vi "LuaVIEW Open.vi"(11 "error in (no error)":errorcluster) -> (6 "LuaVIEW reference":T1, 15 "error out":errorcluster)   [LabVIEW 2012]
doc: "Open a LuaVIEW state that can call public and export functions as well as the other types of LuaVIEW function. The resulting state (passed via the LuaVIEW reference) is ready for script compilation and subsequent execution. Once the LuaVIEW reference is no longer required, close it using \"LuaVIEW Close\" to free the associated resources.\n\nWhen the public function registry is not yet initialized and the \"auto-init registry\" global is set, the registry will be initialized first with all LuaVIEW function VIs in the built executable or, when running under development mode, with all LuaVIEW function VIs in the functions directory of the LuaVIEW toolkit.\n\nNote that the LuaVIEW reference returned by this VI is associated with a new and unique Lua state which entails an instance of the Lua virtual machine as well as the data space involved in compiling scripts and executing the resulting bytecode on that virtual machine instance. Scripts that run on different Lua states therefore have separate variable spaces."
uses:
  typedefs/t_LuaVIEW Reference.ctl
  typedefs/et_LuaVIEW CIN Actions.ctl
  typedefs/t_LuaVIEW CIN Spinlocked Actions.ctl
  glb_LuaVIEW Configuration Globals.vi
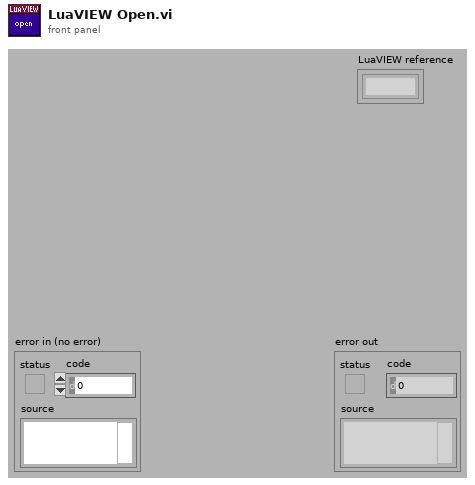
[diagram p1: front panel]
types:
  T1 = typedef "t_LuaVIEW Reference.ctl" = refnum<k1>
  T2 = typedef "et_LuaVIEW CIN Actions.ctl" = enum16{"checksynopsis", "_open", "_registerpublic", "_registerexport", "__never_an_error_result_ns", "luaversion", "cinversion", "_totals", "_taskcount", "pathological", "_unregnextpublic", "registryusecount", "__per_state_actions", "regsetprivate", "regsetindex", "regsetmodule", "_revokeexports", "_usepublic", "prepare", "compile", "execute", "call", "unregstaterefs", "_close", "pullboolean", "pullnumber", "pullI8", "pullU8", "pullI16", "pullU16", "pullI32", "pullU32", "pullobject", "pullrefnum", "pullstring", "pullflat", "pushflat", "pushobject", "getattribute", "setattribute", "stacktostring", "_startyieldtest", "_endyieldtest", "_pollprintbuffer", "__never_an_error_result_ps", "_pollexport", "setclone", "forcecleanup", "gettop", "clearstack", "insert", "pushboolean", "pushnumber", "pushrefnum", "pushstring", "pushnil", "pushvalue", "gettaskref", "settaskref"}
  T3 = typedef "t_LuaVIEW CIN Spinlocked Actions.ctl" = enum16{"totals", "taskcount", "open", "registerpublic", "registerexport", "revokeexports", "unregnextpublic", "usepublic", "pollexport", "close", "startyieldtest", "endyieldtest", "pollprintbuffer"}
  T4 = typedef "et_LuaVIEW CIN Results.ctl" = enum16{"OK", "error", "main", "call", "clonecall", "modulecall", "exportcall", "index", "yield"}
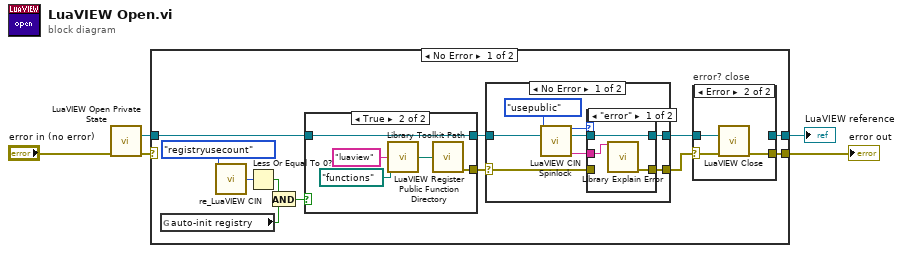
[diagram p0: block diagram]
diagram:
  n1 = call "LuaVIEW Open Private State.vi"("error in (no error)"="error in (no error)") -> ("LuaVIEW reference"=w1:T1, "error out"=w2:errorcluster)  [unwired: 13 in]
  n2 = case shown="No Error" w2 {
    selector: w2 -> [_ w45]
    tunnel: [w17 w44] -> w5
    tunnel: w1 -> [w15 w44]
    tunnel: [w16 w45] -> w4
    frame No Error {
      n3 = global read "glb_LuaVIEW Configuration Globals.vi" "auto-init registry"() -> (w9:bool)
      n4 = call "re_LuaVIEW CIN.vi"("action"=et_LuaVIEW_CIN_Actions."registryusecount") -> ("index out"=w11:i32)  [unwired: 8 in, 6 out]
      n5 = Less Or Equal To 0?(x=w11) -> (x <= 0?=w10:bool)
      n6 = And(x=w10, y=w9) -> (x .and. y?=w8:bool)
      n7 = case shown="True" w8 {
        tunnel: [_ w37] -> w13
        tunnel: w15 -> [w33 w36]
        tunnel: [w33 w36] -> w14
        frame False {
        }
        frame True {
          n8 = call "Library Toolkit Path.vi"("toolkit directory (none)"="luaview", "sub path of toolkit (none)"=path "functions") -> ("absolute toolkit path"=w38:path)  [unwired: 13 in]
          n9 = call "LuaVIEW Register Public Function Directory.vi"("base path"=w38) -> ("error out"=w37:errorcluster)  [unwired: 14 in]
        }
      }
      n10 = case shown="No Error" w13 {
        selector: w13 -> [w18 w32]
        tunnel: [w21 w31] -> w6
        tunnel: [w20 w32] -> w7
        tunnel: w14 -> [w19 w31]
        frame No Error {
          n11 = call "LuaVIEW CIN Spinlock.vi"("action"=t_LuaVIEW_CIN_Spinlocked_Actions."usepublic", "LuaVIEW reference in"=w19) -> ("result"=w24:T4, "LuaVIEW reference out"=w23:T1, "string out"=w22:string)  [unwired: 7 in, 4 out]
          n12 = case shown="\"error\"" w24 {
            tunnel: w22 -> [w26 _]
            tunnel: [w28 w29] -> w20
            tunnel: w23 -> [w27 w30]
            tunnel: [w27 w30] -> w21
            tunnel: w18 -> [_ w29]
            frame "error" {
              n13 = call "Library Explain Error.vi"("explanation prefix (none)"=w26) -> ("explained error"=w28:errorcluster)  [unwired: 14 in]
            }
            frame Default {
            }
          }
        }
        frame Error {
        }
      }
      n14 = case "error? close" shown="Error" w7 {
        selector: w7 -> [w39 w42]
        tunnel: w6 -> [w40 w43]
        tunnel: [w40 _] -> w17
        tunnel: [w39 w41] -> w16
        frame No Error {
        }
        frame Error {
          n15 = call "LuaVIEW Close.vi"("LuaVIEW reference"=w43, "error in (no error)"=w42) -> ("dup error"=w41:errorcluster)  [unwired: 13 in]
        }
      }
    }
    frame Error {
    }
  }
  "LuaVIEW reference" <- w5
  "error out" <- w4
